vi "Build core.vi"(6 "Previous Build's Artifacts":refnum<class "Build Artifact.lvclass">[](array[class]), 7 "Progress":refnum<class "Progress.lvclass">, 8 "error in (no error)":errorcluster, 10 "Build Cache":refnum<class "Build Cache.lvclass">, 11 "Build Item in":refnum<class "Build VIPB Step.lvclass">) -> (0 "error out":errorcluster, 1 "Explore Path":path, 2 "Build Results":T1, 4 "New Artifacts":refnum<class "Build Artifact.lvclass">[](array[class]))   [LabVIEW 2019, in "VIPM.lvlib" / "Build VIPB Step.lvclass"]
doc: "Performs all the necessary build actions for the build step.\n\nCopyright: MGI 2016\nAuthor: Derek Trepanier"
uses:
  Build VIPB Step.lvclass
  libs/Solution.lvlibp/Solution/Progress/Progress.lvclass
  libs/Solution.lvlibp/Solution/Build Artifact/Build Artifact.lvclass
  libs/Solution.lvlibp/Solution/Build Item/Build Result.ctl
  libs/Solution.lvlibp/Solution/Build Cache/Build Cache.lvclass
  Build VIPB Step.lvclass/Build VIPB Step.ctl
  libs/Project.lvlibp/Project/Binary File/Binary File.lvclass
  C:/Users/pasca/source/repos/mgi-solution-explorer-extensions/libs/Solution.lvlibp/Solution/Build Artifact/Build Artifact.lvclass
  <vilib>/JKI/VIPM API/VIPM API_vipm_api.lvlib
  libs/Solution.lvlibp/Solution/Build Item/Build Step.lvclass
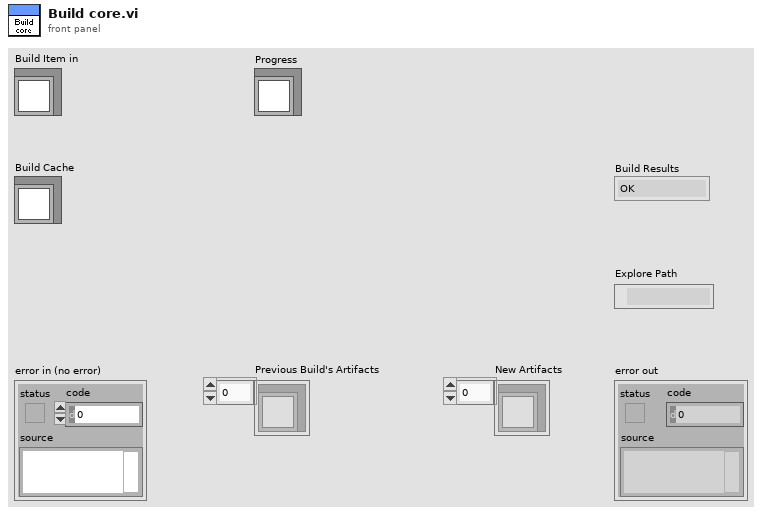
[diagram p1: front panel]
types:
  T1 = typedef "Solution.lvlibp/Build Step.lvclass/Build Result.ctl" = enum16{"OK", "Skipped", "Error"}
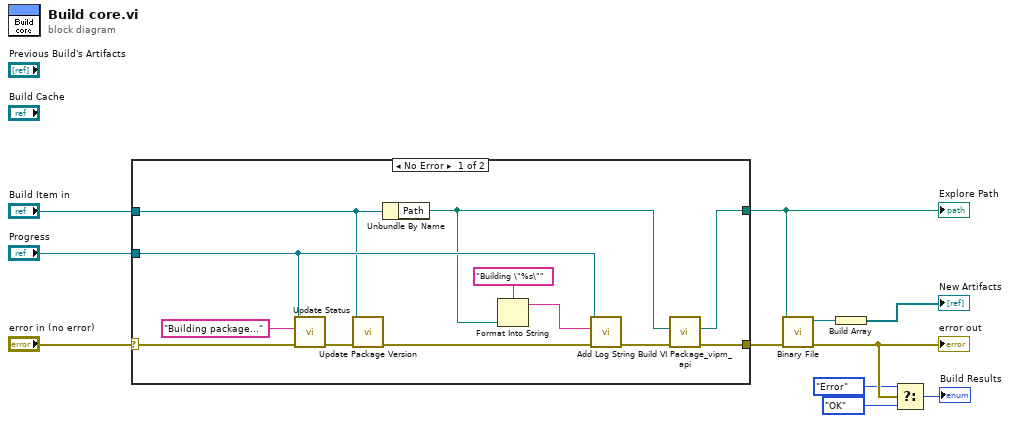
[diagram p0: block diagram]
diagram:
  n1 = case shown="No Error" "error in (no error)" {
    selector: "error in (no error)" -> [w23 w24]
    tunnel: [w16 w24] -> w10
    tunnel: [w17 _] -> w9
    tunnel: "Build Item in" -> [w12 _]
    tunnel: "Progress" -> [w21 _]
    frame No Error {
      n2 = call "Update Status.vi"("error in (no error)"=w23, "Status String"="Building package...", "Progress in"=w21) -> ("error out"=w15:errorcluster)  [unwired: 8 in]
      n3 = call "Update Package Version.vi"("error in (no error)"=w15, "Build Package Step in"=w12) -> ("error out"=w14:errorcluster)  [unwired: 8 in, 1 out]
      n4 = Unbundle By Name(w12) -> ("Path"=w18:path)
      n5 = Format Into String(format string="Building \"%s\"" ("Log Item"), w18) -> (resulting string=w20:string)  [unwired: 2 in, 1 out]
      n6 = call "Add Log String.vi"("error in (no error)"=w14, "Log Item"=w20, "Progress in"=w21) -> ("error out"=w13:errorcluster)  [unwired: 8 in]
      n7 = call <vilib>:"Build VI Package_vipm_api.vi"("error in (no error)"=w13, "Path to VIPB File"=w18) -> ("error out"=w16:errorcluster, "Build Output"=w17:path)  [unwired: 8 in]
    }
    frame Error {
    }
  }
  "Explore Path" <- w9
  n8 = call "Binary File.vi"("error in (no error)"=w10, "File"=w9) -> ("error out"=w3:errorcluster, "Binary File out"=w8:refnum<class "Binary File.lvclass">)  [unwired: 8 in]
  "error out" <- w3
  n9 = Build Array(w8) -> (→"New Artifacts":refnum<class "Binary File.lvclass">[])
  n10 = Select(t=Build_Result."Error" ("Build Results"), s=w3, f=Build_Result."OK" ("Build Results")) -> (s? t:f=→"Build Results":T1)
